vi "DEBUG Hoverボタン.vi"() -> ()   [LabVIEW 2014]
uses:
  <vilib>/Utility/cursorutil.llb/Set Cursor (Icon Pict).vi
panel:
  in  "OKボタン 3":bool
  in  "停止":bool
  in  "OKボタン 2":bool
  in  "OKボタン":bool
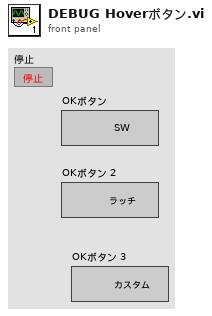
[diagram p1: front panel]
types:
  T1 = cluster{"OFF色":cluster{u32, u32}, "ON色":cluster{u32, u32}, "ONOFF":cluster{u32, u32}, "OFFON":cluster{u32, u32}}
  T2 = cluster{"通常ボタン色":cluster{u32, u32}[], "HOVER色":cluster{"Color":u32, "Color":u32}[]}
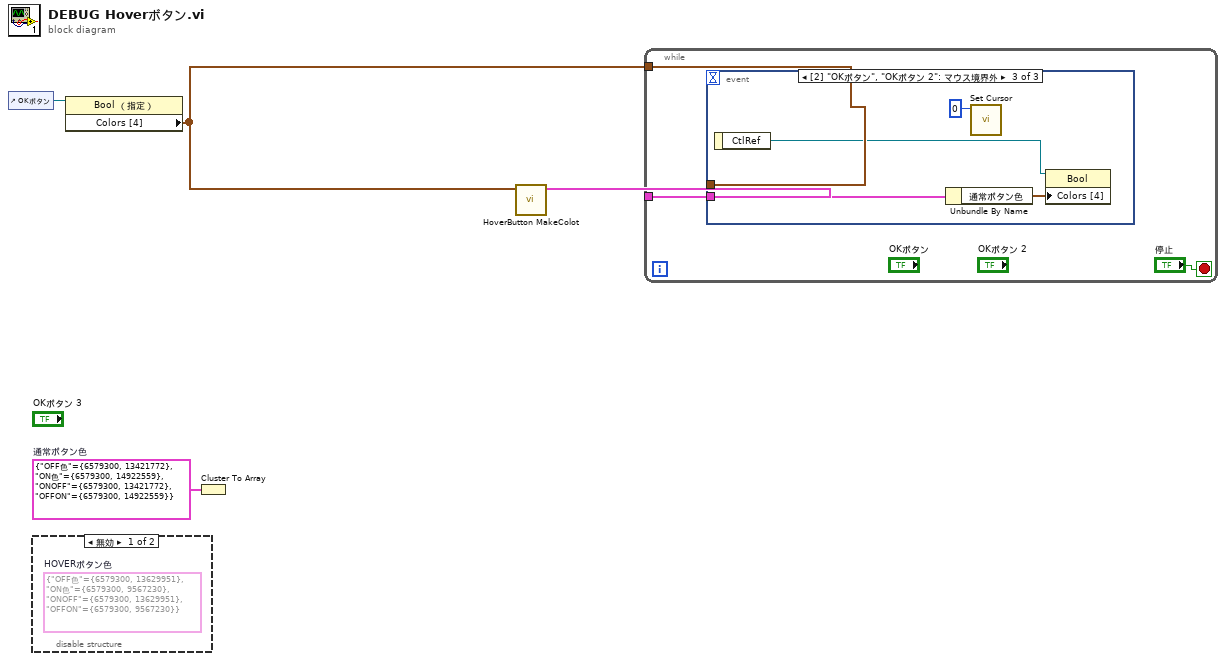
[diagram p0: block diagram]
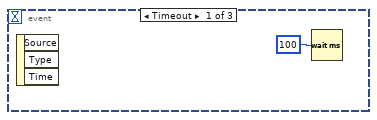
[diagram p3: hidden frame]
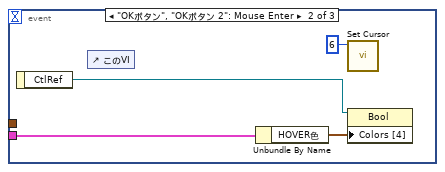
[diagram p4: hidden frame]
diagram:
  w2 = T1 {"OFF色"={6579300, 13421772}, "ON色"={6579300, 14922559}, "ONOFF"={6579300, 13421772}, "OFFON"={6579300, 14922559}}  # 通常ボタン色
  n1 = control-ref of="OKボタン"() -> (w4:refnum<vi>)
  n2 = disable-structure shown="無効" {
    frame Disabled {
      (unwired) T1 {"OFF色"={6579300, 13629951}, "ON色"={6579300, 9567230}, "ONOFF"={6579300, 13629951}, "OFFON"={6579300, 9567230}}  # HOVERボタン色
    }
    frame Enabled {
    }
  }
  n3 = property class="Bool （指定）"(reference=w4) -> ("Colors [4]"=w1:cluster{u32, u32}[])  [unwired: 1 in, 2 out]
  n4 = Cluster To Array(cluster=w2) -> ()  [unwired: 1 out]
  n5 = call "HoverButton MakeColot.vi"("Colors [4]"=w1) -> ("クラスタ"=w3:T2)  [unwired: 10 in]
  n6 = while {
    tunnel: w3 -> [w6]
    tunnel: w1 -> [w5]
    stop <- "停止" stop-if-true
    n7 = event shown="[2] \"OKボタン\", \"OKボタン 2\": マウス境界外" {
      selector: _ -> [_ _ _]
      dyn-events: _ -> [_ _ _]
      timeout: _ -> [_ _ _]
      tunnel: w5 -> [_ _ _]
      tunnel: w6 -> [_ w11 w15]
      event Timeout {
        n8 = event-data() -> ()  [unwired: 1 in, 3 out]
        n9 = Wait (ms)(milliseconds to wait=u32 100 ("ミリ秒待機時間")) -> ()  [unwired: 1 out]
      }
      event "OKボタン", "OKボタン 2": Mouse Enter {
        n10 = event-data() -> ("CtlRef"=w12:refnum<vi>)  [unwired: 1 in]
        n11 = control-ref of="このVI"() -> ()  [unwired: 1 out]
        n12 = Unbundle By Name(w11) -> ("HOVER色"=w10:cluster{"Color":u32, "Color":u32}[])
        n13 = call-poly <vilib>:"Set Cursor.vi"("icon"=u16 6) -> ()  [unwired: 9 in, 2 out]
        n14 = property class="Bool"(reference=w12, "Colors [4]"=w10) -> ()  [unwired: 1 in, 2 out]
      }
      event "OKボタン", "OKボタン 2": Mouse Leave {
        n15 = event-data() -> ("CtlRef"=w16:refnum<vi>)  [unwired: 1 in]
        n16 = Unbundle By Name(w15) -> ("通常ボタン色"=w14:cluster{u32, u32}[])
        n17 = call-poly <vilib>:"Set Cursor.vi"("icon"=u16 0) -> ()  [unwired: 9 in, 2 out]
        n18 = property class="Bool"(reference=w16, "Colors [4]"=w14) -> ()  [unwired: 1 in, 2 out]
      }
    }
  }
